vi "Reading Value.vi"(10 "Result Refnum":refnum<vi>, 11 "Measure":T1) -> (1 "Exit!":T1, 2 "Go to Idle":T1, 3 "Measure":T1)   [LabVIEW 2017]
uses:
  <extravilib>/ChannelInstances/Messenger-bool/))Channel.ctl
  <extravilib>/ChannelInstances/Messenger-bool/Read With Abort.vi
  <extravilib>/ChannelInstances/Messenger-bool/Write With Abort.vi
  <resource>/Channels/Messenger/Read With Abort.vi
  <vilib>/ChannelSupport/Channel Message/Read ID.vi
  <resource>/Channels/Messenger/Write With Abort.vi
  <extravilib>/ChannelInstances/Messenger-bool/Wrapper.lvclass
  C:/Program Files (x86)/National Instruments/LabVIEW 2017/vi.lib/ChannelSupport/Channel Message/Channel Message.lvclass
  <resource>/Channels/Messenger/Endpoint.vi
  <extravilib>/ChannelInstances/Messenger-bool/Unwrap.vi
  <extravilib>/ChannelInstances/Messenger-bool/Wrap.vi
  <extravilib>/ChannelInstances/Messenger-bool.lvlib
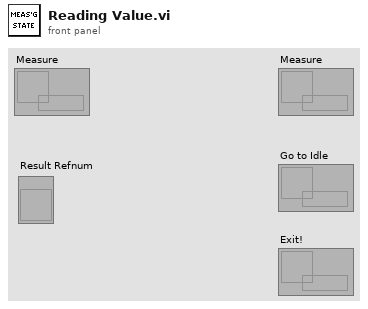
[diagram p1: front panel]
types:
  T1 = typedef "Messenger-bool.lvlib/))Channel.ctl" = refnum<queue>
  T2 = enum16{"Left Button", "Center Button", "Right Button", "Window Close"}
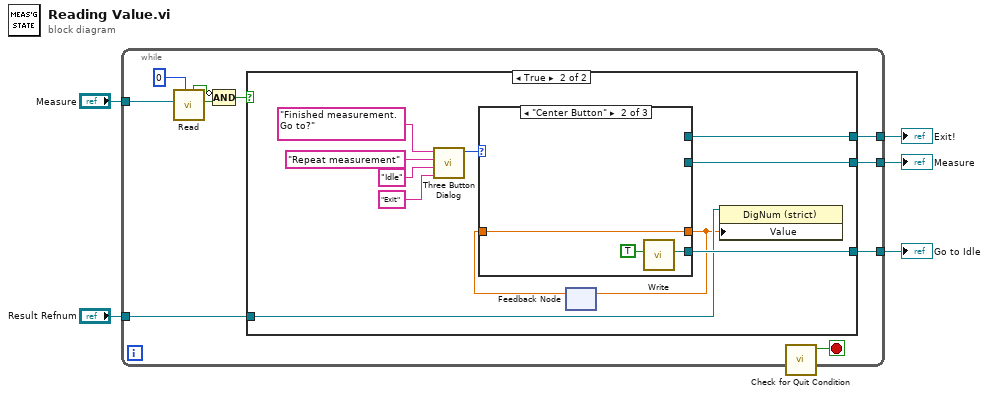
[diagram p0: block diagram]
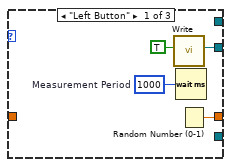
[diagram p3: hidden frame]
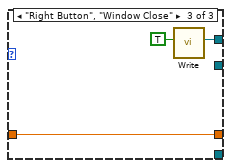
[diagram p4: hidden frame]
diagram:
  n1 = while {
    tunnel: "Measure" -> [w15]
    tunnel: [w14] -> w4
    tunnel: [w13] -> w3
    tunnel: [w12] -> w2
    tunnel: "Result Refnum" -> [w6]
    stop <- w7 stop-if-true
    n2 = call <extravilib>:"Read.vi"("timeout in ms (-1)"=0, "channel"=w15) -> ("element"=w9:bool, "timedout?"=w10:bool)  [unwired: 6 in, 2 out]
    n3 = Compound Arithmetic op=AND(invert w10, w9) -> (w8:bool)
    n4 = case shown="True" w8 {
      tunnel: [_ w21] -> w14
      tunnel: [_ w20] -> w13
      tunnel: [_ w19] -> w12
      tunnel: w6 -> [_ w17]
      frame False {
      }
      frame True {
        n5 = call <vilib>:"Three Button Dialog.vi"("Right Button Text (\"Cancel\")"="Exit" ("Right Button Text (\"Cancel\")"), "Center Button Text (\"No\")"="Idle" ("Center Button Text (\"No\")"), "Left Button Text (\"Yes\")"="Repeat measurement" ("Left Button Text (\"Yes\")"), "message"="Finished measurement. Go to?") -> ("Which Button?"=w22:T2)  [unwired: 7 in]
        n6 = feedback #1() -> (w18:dbl)  [unwired: 1 in]
        n7 = case shown="\"Center Button\"" w22 {
          tunnel: [_ _ w35] -> w21
          tunnel: [w29 _ _] -> w20
          tunnel: [_ w32 _] -> w19
          tunnel: [w27 w31 w34] -> w16
          tunnel: w18 -> [_ w31 w34]
          frame "Left Button" {
            w28 = u32 1000  # Measurement Period
            n8 = call <extravilib>:"Write.vi"("element"=TRUE) -> ("channel"=w29:T1)  [unwired: 8 in, 2 out]
            n9 = Wait (ms)(milliseconds to wait=w28) -> ()  [unwired: 1 out]
            n10 = Random Number (0-1)() -> (number: 0 to 1=w27:dbl)
          }
          frame "Center Button" {
            n11 = call <extravilib>:"Write.vi"("element"=TRUE) -> ("channel"=w32:T1)  [unwired: 8 in, 2 out]
          }
          frame "Right Button", "Window Close" {
            n12 = call <extravilib>:"Write.vi"("element"=TRUE) -> ("channel"=w35:T1)  [unwired: 8 in, 2 out]
          }
        }
        n13 = feedback-in #1(w16) -> ()
        n14 = property class="DigNum (strict)"(reference=w17, "Value"=w16) -> ()  [unwired: 1 in, 2 out]
      }
    }
    n15 = call "Check for Quit Condition.vi"() -> ("Quit?"=w7:bool)  [unwired: 11 in]
  }
  "Exit!" <- w4
  "Measure" <- w3
  "Go to Idle" <- w2
